vi "decimate_waveforms.vi"(8 "error in (no error)":errorcluster, 11 "LockinDAQ":refnum<class "Instrument.DAQ.lvclass">) -> (0 "error out":errorcluster, 3 "LockinDAQ out":refnum<class "Instrument.DAQ.lvclass">)   [LabVIEW 2019, in "Instrument.DAQ.lvclass"]
doc: "Decimates the input sequence X by the decimating factor and the averaging Boolean control."
uses:
  Instrument.DAQ.lvclass
  Instrument.DAQ.lvclass/Instrument.DAQ.ctl
  <vilib>/Analysis/2dsp.llb/Decimate (single shot, DBL).vi
  <vilib>/Waveform/WDTOps.llb/WDT Number of Waveform Samples DBL.vi
  <vilib>/Analysis/NI_AALPro.lvlib
  <vilib>/addons/Digital Filter Design/NI_DigFilterLicensed.lvlib
  <vilib>/addons/Digital Filter Design/_Objects.llb/DFD Multirate Filtering Mode.ctl
  <vilib>/measure/NI_MABase.lvlib
  <vilib>/addons/Digital Filter Design/_Objects.llb/DFD Multirate Filter Specification (Design).ctl
  <vilib>/addons/Digital Filter Design/Design.llb/DFD MRate Filter Design (Integer).vi
  <vilib>/addons/Digital Filter Design/Multirate.llb/DFD MRate Filtering (Wfm NChan).vi
  <vilib>/addons/Digital Filter Design/Multirate.llb/DFD NStage MRate Filtering (Wfm).vi
panel:
  out "x-y":dbl
  out "fs/2M":dbl
  in  "fpass":dbl
  in  "amplitude":dbl=1.0 format="%0.2p"
  in  "frequency":dbl=10.0 format="%0.2p"
  in  "sampling info":cluster{"Fs":dbl, "#s":dbl}={"Fs"=1000.0, "#s"=10000.0}
  out "x/y":dbl
  in  "decimation":i32=4
  out "# samples 2":i32
  out "# samples 1":i32
  # "by Marco Tedaldi, Brain Research Institute, University of Zurich, 2013"
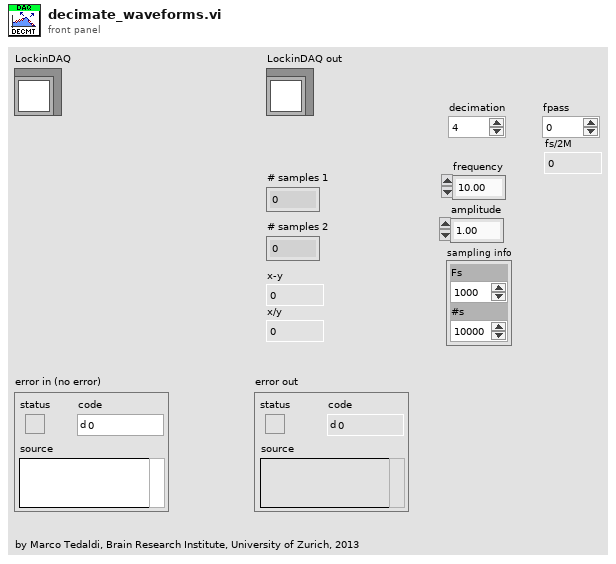
[diagram p1: front panel]
types:
  T1 = typedef "Instrument.DAQ.lvclass/PublicEvents--DAQ.getWaveforms.ctl" = cluster{"AO":waveform(dbl)[], "AI":waveform(dbl)[], "RefX":waveform(dbl)[], "RefY":waveform(dbl)[]}
  T2 = typedef "NI_DigFilterLicensed.lvlib/DFD Multirate Filter Specification (Design).ctl" = cluster{"fpass":dbl, "fstop":dbl}
  T3 = typedef "NI_DigFilterLicensed.lvlib/DFD Multirate Filtering Mode.ctl" = u16
  T4 = typedef "NI_DigFilterLicensed.lvlib/DFD Multirate Filter Obj.ctl" = cluster{"mMRate_Structure":enum16{"CIC", "FIR", "IIR", "Lattice"}, "mMRate_Mode":T5, "mMRate_Factor":i32, "mMRate_FIRParams":cluster{"mMRate_FIR_H":dbl[], "mMRate_FIR_IsNyquist?":bool, "mMRate_FIR_IsSymmetric?":bool}, "mMRate_CICParams":cluster{"mMRate_CIC_#Stage":i32, "mMRate_CIC_Lag":i32, "mMRate_CIC_Type":enum16{"Lowpass", "Highpass"}}, "mMRate_Order":i32, "mMRate_Version":string, "mMRate_Comments":string, "mMRate_RationalFactor":cluster{"mMRate_L":i32, "mMRate_M":i32}, "mMRate_Fs":dbl, "mMRate_Quantized?":bool, "mMRate_QFilterGain":dbl, "mMRate_CoefWl":i16, "mMRate_Scaling":cluster{"mMRate_ScaleByPowerOf2?":bool, "mMRate_ScaleType":T6}, "mMRate_InputWl":i16, "mMRate_OutputWl":i16, "mMRate_OutputMode":T7, "mMRate_MultMode":T8, "mMRate_BitPruning":bool, "mMRate_GainWl":i16, "mMRate_OutputFwl":i16, "mMRate_SumIwl":i16, "mMRate_InputIwl ":i16, "mMRate_SumWl":i16, "mMRate_CoefIwl":i16}
  T5 = typedef "NI_DigFilterLicensed.lvlib/DFD Multirate Mode.ctl" = i16
  T6 = typedef "NI_DigFilterLicensed.lvlib/DFD Coef Norm Type.ctl" = enum16{"No Norm", "Time Domain 1-Norm", "Time Domain 2-Norm", "Time Domain Inf-Norm"}
  T7 = typedef "NI_DigFilterLicensed.lvlib/DFD Round-off Mode.ctl" = enum16{"Nearest", "Truncation"}
  T8 = typedef "NI_DigFilterLicensed.lvlib/DFD FXP MRate Multiply Mode.ctl" = enum16{"Truncated", "Full"}
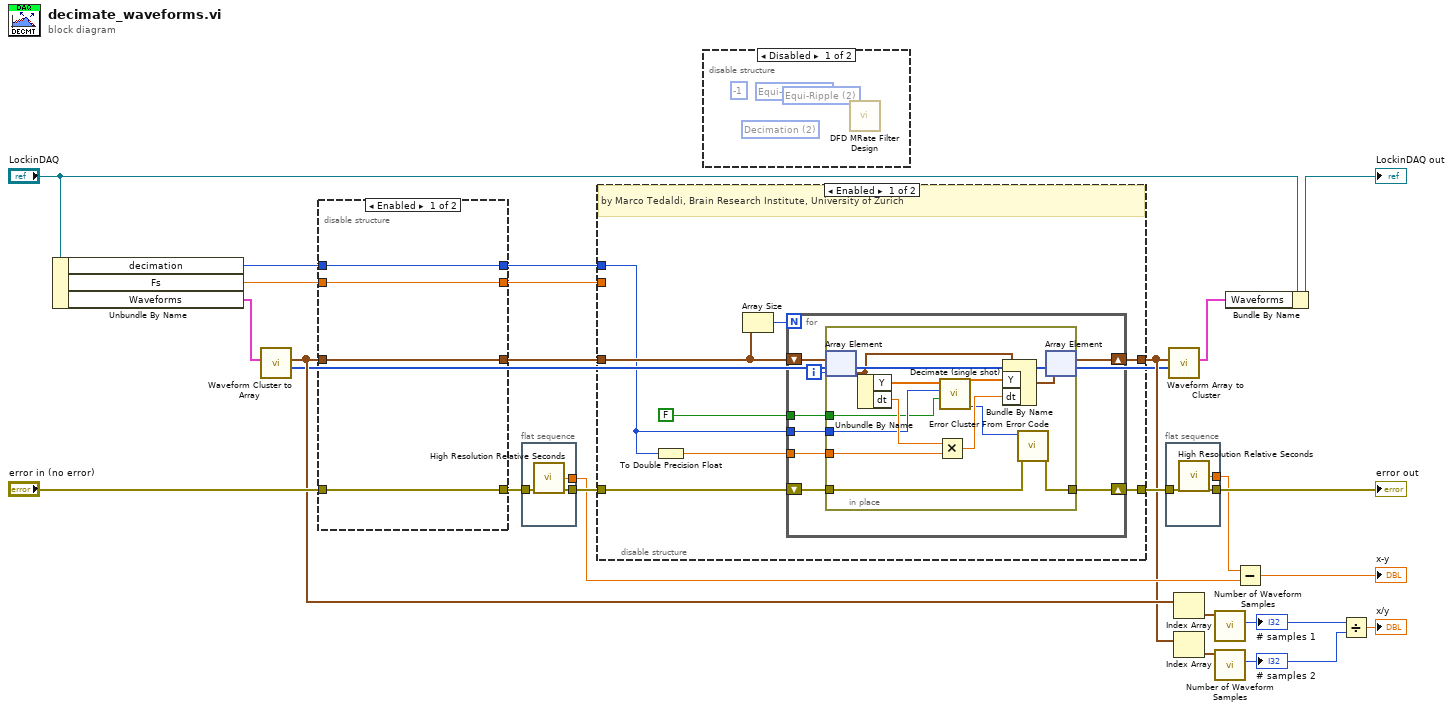
[diagram p0: block diagram]
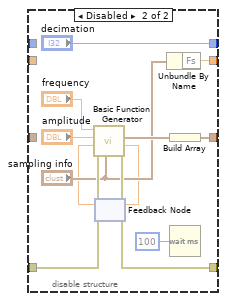
[diagram p2: hidden frame]
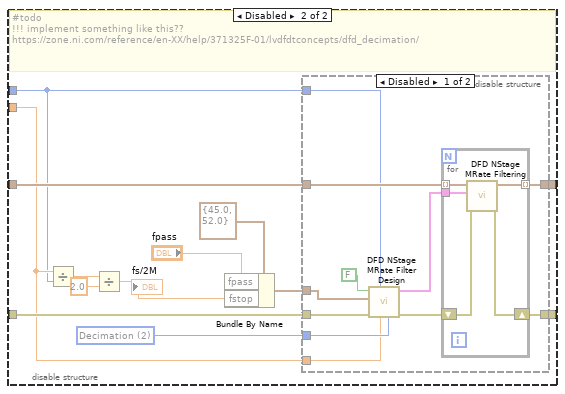
[diagram p4: hidden frame]
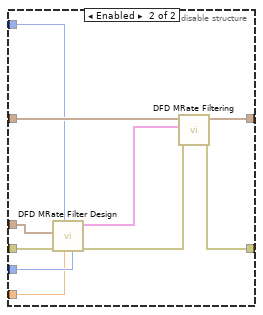
[diagram p5: hidden frame]
diagram:
  n1 = Unbundle By Name("LockinDAQ") -> ("decimation"=w21:u32, "Fs"=w23:dbl, "Waveforms"=w7:T1)
  n2 = call "Waveform Cluster to Array.vi"("Waveform Cluster"=w7) -> ("Lengths"=w1:i32[], "Concatenated Waveforms"=w4:waveform(dbl)[])  [unwired: 9 in]
  n3 = disable-structure shown="Enabled" {
    disable-tunnel: [w29 w40] -> w24
    disable-tunnel: w23 -> [w29 _]
    disable-tunnel: [w28 "decimation"] -> w22
    disable-tunnel: w21 -> [w28 _]
    disable-tunnel: w4 -> [w27 _]
    disable-tunnel: [w27 w30] -> w19
    disable-tunnel: "error in (no error)" -> [w26 w35]
    disable-tunnel: [w26 w34] -> w9
    frame Enabled {
    }
    frame Disabled {
      n4 = feedback #1() -> (w32:dbl)  [unwired: 1 in]
      n5 = call <vilib>:"Basic Function Generator.vi"("sampling info"="sampling info", "error in (no error)"=w35, "phase"=w32, "amplitude"="amplitude", "frequency"="frequency") -> ("error out"=w34:errorcluster, "phase out"=w31:dbl, "signal out"=w39:waveform(dbl))  [unwired: 4 in]
      n6 = feedback-in #1(w31) -> ()
      n7 = Unbundle By Name("sampling info") -> ("Fs"=w40:dbl)
      n8 = Build Array(w39) -> (w30:waveform(dbl)[])
      n9 = Wait (ms)(milliseconds to wait=u32 100) -> ()  [unwired: 1 out]
    }
  }
  n10 = flat-sequence {
    tunnel: [w43] -> w18
    tunnel: w9 -> [w43]
    tunnel: [w42] -> w16
    frame #0 {
      n11 = call <vilib>:"High Resolution Relative Seconds.vi"() -> ("relative seconds"=w42:dbl)
    }
  }
  n12 = disable-structure shown="Enabled" {
    disable-tunnel: w18 -> [w45 w81]
    disable-tunnel: [w49 w82] -> w3
    disable-tunnel: [w46 w84] -> w25
    disable-tunnel: w19 -> [w48 w83]
    disable-tunnel: w22 -> [w47 w76]
    disable-tunnel: w24 -> [_ w79]
    frame Enabled {
      # "by Marco Tedaldi, Brain Research Institute, University of Zurich"
      n13 = To Double Precision Float(number=w47) -> (double precision float=w51:dbl)
      n14 = Array Size(array=w48) -> (size(s)=w44:i32)
      n15 = for {
        N: w44 -> [_]
        tunnel: w51 -> [w59]
        tunnel: w47 -> [w58]
        tunnel: FALSE ("averaging") -> [w57]
        shift-right: [w53] -> w49
        shift-left: w48 -> [w55]
        shift-right: [w56] -> w46
        shift-left: w45 -> [w52]
        i -> [w54]
        n16 = in-place {
          in-place-border: w59 -> [w68]
          in-place-border: w58 -> [w67]
          in-place-border: w57 -> [w65]
          in-place-border: [w60] -> w56
          in-place-border: w52 -> [w61]
          n17 = in-place-array #2(w55, w54) -> (w62:waveform(dbl))
          n18 = Unbundle By Name(w62) -> ("Y"=w71:dbl[], "dt"=w69:dbl)
          n19 = Multiply(x=w69, y=w68) -> (x*y=w66:dbl)
          n20 = call-poly <vilib>:"Decimate (single shot).vi"("averaging"=w65, "decimating factor"=w67, "X"=w71) -> ("error"=w64:i32, "Decimated Array"=w70:dbl[])  [unwired: 7 in]
          n21 = Bundle By Name(cluster=w62, "Y"=w70, "dt"=w66) -> (w63:waveform(dbl))
          n22 = call <vilib>:"Error Cluster From Error Code.vi"("error in (no error)"=w61, "error code (0)"=w64) -> ("error out"=w60:errorcluster)  [unwired: 7 in]
          n23 = in-place-array #2(w63) -> (w53:waveform(dbl)[])  [unwired: 1 out]
        }
      }
    }
    frame Disabled {
      w80 = T3 2 items=["No Rate Change", "Interpolation", "Decimation"] ("filtering mode")
      # "#todo\n!!! implement something like this??\nhttps://zone.ni.com/reference/en-XX/help/371325F-01/lvdfdtconcepts/dfd_decimation/"
      n24 = Divide(x=w79, y=w76) -> (x/y=w75:dbl)
      n25 = Divide(x=w75, y=2.0) -> (x/y=w73:dbl)
      "fs/2M" <- w73
      n26 = Bundle By Name(cluster=T2 {"fpass"=45.0, "fstop"=52.0} ("freq specs [Hz]"), "fpass"="fpass", "fstop"=w73) -> (w72:T2)
      n27 = disable-structure shown="Disabled" {
        disable-tunnel: [w95 w102] -> w84
        disable-tunnel: w83 -> [w94 w106]
        disable-tunnel: [w93 w104] -> w82
        disable-tunnel: w81 -> [w92 w110]
        disable-tunnel: w80 -> [w90 w108]
        disable-tunnel: w79 -> [w87 w107]
        disable-tunnel: w76 -> [w86 w101]
        disable-tunnel: w72 -> [w85 w109]
        frame Disabled {
          n28 = call <vilib>:"DFD NStage MRate Filter Design.vi"("filtering mode"=w90, "fs in [Hz]"=w87, "factor"=w86, "error in (no error)"=w92, "freq specs [Hz]"=w85, "using CIC?"=FALSE) -> ("error out"=w91:errorcluster, "multirate filters out"=w89:T4[])  [unwired: 4 in]
          n29 = for {
            tunnel: w94 -> [w98] mode=indexing
            tunnel: [w97] -> w93 mode=indexing
            tunnel: w89 -> [w96]
            shift-right: [w100] -> w95
            shift-left: w91 -> [w99]
            n30 = call-poly <vilib>:"DFD NStage MRate Filtering.vi"("error in (no error)"=w99, "multirate filters"=w96, "signal in"=w98) -> ("error out"=w100:errorcluster, "signal out"=w97:waveform(dbl))  [unwired: 7 in]
          }
        }
        frame Enabled {
          n31 = call-poly <vilib>:"DFD MRate Filter Design.vi"("filtering mode"=w108, "fs in [Hz]"=w107, "factor"=w101, "error in (no error)"=w110, "freq specs [Hz]"=w109) -> ("error out"=w103:errorcluster, "multirate filter out"=w105:T4)  [unwired: 5 in]
          n32 = call-poly <vilib>:"DFD MRate Filtering.vi"("error in (no error)"=w103, "multirate filter"=w105, "signal in"=w106) -> ("error out"=w102:errorcluster, "signal out"=w104:waveform(dbl)[])  [unwired: 7 in]
        }
      }
    }
  }
  n33 = disable-structure shown="Disabled" {
    frame Disabled {
      (unwired) -1 ("order")
      (unwired) u16 2 items=["Kaiser Window", "Dolph-Chebyshev Window", "Equi-Ripple"] ("method")
      w111 = u16 2 items=["Kaiser Window", "Dolph-Chebyshev Window", "Equi-Ripple"] ("method")
      (unwired) T3 2 items=["No Rate Change", "Interpolation", "Decimation"] ("filtering mode")
      n34 = call-poly <vilib>:"DFD MRate Filter Design.vi"() -> ()  [unwired: 10 in, 2 out]
    }
    frame Enabled {
    }
  }
  n35 = flat-sequence {
    tunnel: [w113] -> w17
    tunnel: w25 -> [w113]
    tunnel: [w112] -> w8
    frame #0 {
      n36 = call <vilib>:"High Resolution Relative Seconds.vi"() -> ("relative seconds"=w112:dbl)
    }
  }
  n37 = call "Waveform Array to Cluster.vi"("Lengths"=w1, "Concatenated Waveforms"=w3) -> ("Waveform Cluster"=w2:T1)  [unwired: 9 in]
  n38 = Index Array(array=w4) -> (element=w14:waveform(dbl))  [unwired: 1 in]
  n39 = Index Array(array=w3) -> (element=w13:waveform(dbl))  [unwired: 1 in]
  n40 = call-poly <vilib>:"Number of Waveform Samples.vi"("waveform in"=w14) -> ("number of samples"=w5:i32)  [unwired: 8 in, 2 out]
  "# samples 1" <- w5
  n41 = call-poly <vilib>:"Number of Waveform Samples.vi"("waveform in"=w13) -> ("number of samples"=w6:i32)  [unwired: 8 in, 2 out]
  "# samples 2" <- w6
  n42 = Bundle By Name(cluster="LockinDAQ", "Waveforms"=w2) -> (→"LockinDAQ out":refnum<class "Instrument.DAQ.lvclass">)
  n43 = Subtract(x=w8, y=w16) -> (x-y=→"x-y":dbl)
  n44 = Divide(x=w5, y=w6) -> (x/y=→"x/y":dbl)
  "error out" <- w17
